vi "Get Value.vi"(8 "error in (no error)":errorcluster, 11 "Ctrl Reference's in":refnum<class "Ctrl Reference's.lvclass">) -> (0 "error out":errorcluster, 1 "Not Empty Value?":bool, 2 "Value Out":variant, 3 "Ctrl Reference's out":refnum<class "Ctrl Reference's.lvclass">, 4 "Ctl Refnum":refnum<vi>)   [LabVIEW 2023, in "Ctrl Reference's.lvclass"]
uses:
  Ctrl Reference's.lvclass
  Ctrl Reference's.lvclass/Ctrl Reference's.ctl
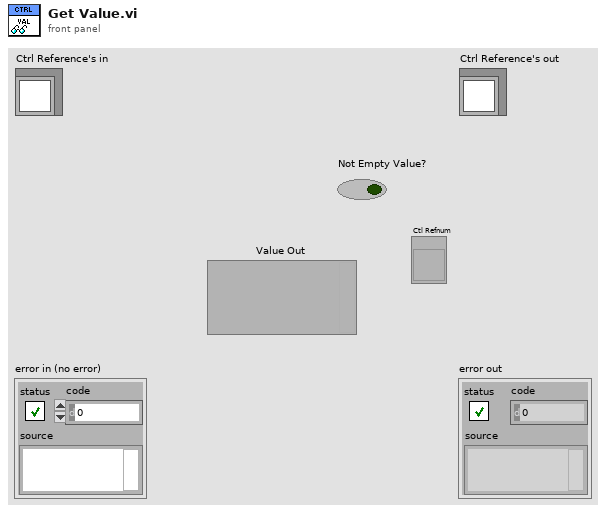
[diagram p1: front panel]
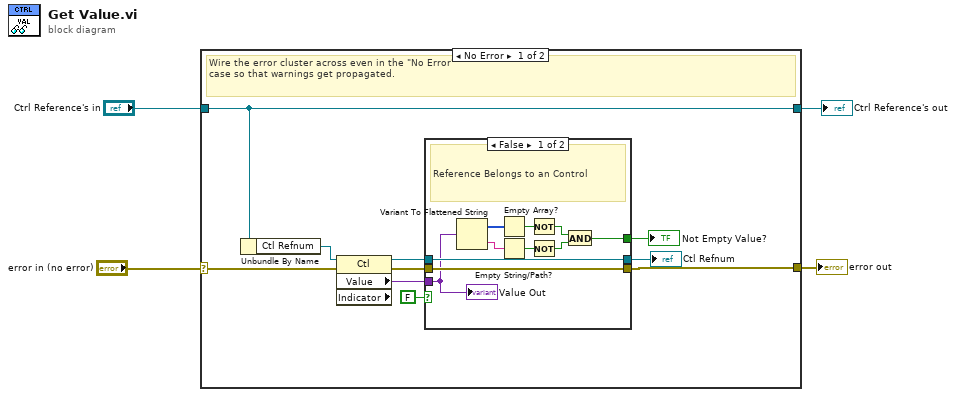
[diagram p0: block diagram]
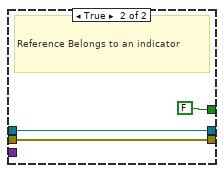
[diagram p2: hidden frame]
diagram:
  n1 = case shown="No Error" "error in (no error)" {
    selector: "error in (no error)" -> [w9 w29]
    tunnel: [w7 w29] -> w3
    tunnel: [w10 w28] -> w1
    tunnel: "Ctrl Reference's in" -> [w10 w28]
    frame No Error {
      # "Wire the error cluster across even in the \"No Error\"\ncase so that warnings get propagated."
      n2 = Unbundle By Name(w10) -> ("Ctl Refnum"=w8:refnum<vi>)
      n3 = property class="Ctl" props=["Value", "Indicator"](reference=w8, error in=w9) -> (reference out=w14:refnum<vi>, error out=w13:errorcluster, "Value"=w12:variant)  [unwired: 1 out]
      n4 = case shown="False" FALSE {
        tunnel: [w24 w27] -> w5
        tunnel: w14 -> [w24 w27]
        tunnel: w13 -> [w23 w26]
        tunnel: [w23 w26] -> w7
        tunnel: w12 -> [w15 _]
        tunnel: [w16 FALSE] -> w11
        frame False {
          # "Reference Belongs to an Control"
          n5 = Variant To Flattened String(Variant=w15) -> (data string=w21:string, 1:w22:i16[])
          n6 = Empty Array?(array=w22) -> (empty?=w20:bool)
          n7 = Empty String/Path?(string/path=w21) -> (empty?=w19:bool)
          n8 = Not(x=w20) -> (.not. x?=w18:bool)
          n9 = Not(x=w19) -> (.not. x?=w17:bool)
          n10 = And(x=w18, y=w17) -> (x .and. y?=w16:bool)
          "Value Out" <- w15
        }
        frame True {
          # "Reference Belongs to an indicator"
        }
      }
      "Not Empty Value?" <- w11
      "Ctl Refnum" <- w5
    }
    frame Error {
    }
  }
  "error out" <- w3
  "Ctrl Reference's out" <- w1
